vi "set parameter - i8.vi"(8 "error in (no error)":errorcluster, 9 "value":i8, 10 "parameter":u8 format="%x", 11 "channel":u16 format="%x") -> (0 "error out":errorcluster)   [LabVIEW 2024, in "atsj peakcan basic.lvlib"]
doc: "Sets a parameter for a PeakCAN <b>channel</b>."
uses:
  atsj peakcan basic.lvlib
  support/x64/PCANBasic.dll
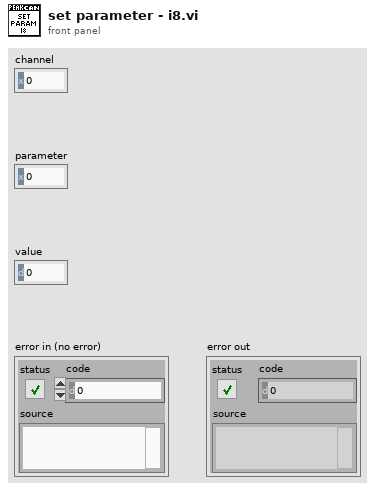
[diagram p1: front panel]
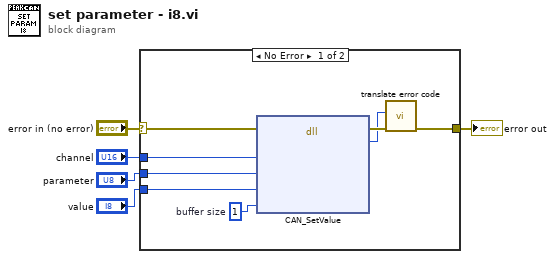
[diagram p0: block diagram]
diagram:
  n1 = case shown="No Error" "error in (no error)" {
    selector: "error in (no error)" -> [w10 w14]
    tunnel: [w9 w14] -> w4
    tunnel: "channel" -> [w8 _]
    tunnel: "parameter" -> [w7 _]
    tunnel: "value" -> [w6 _]
    frame No Error {
      w13 = u16 1  # buffer size
      n2 = dll-call lib="C:/atsj/plateau/atsj-peakcan-basic-for-labview/src/support/x64/PCANBasic.dll" fn="CAN_SetValue" ("set parameter - i8")(error in=w10, "Channel"=w8, "Parameter"=w7, "Buffer"=w6, "BufferLength"=w13) -> (error out=w12:errorcluster, "Status"=w11:u32)  [unwired: 6 in, 1 out]
      n3 = call "translate error code.vi"("error in (no error)"=w12, "error code"=w11) -> ("error out"=w9:errorcluster)  [unwired: 9 in]
    }
    frame Error {
    }
  }
  "error out" <- w4
